vi "Write Header and Footer [ ].vi"(8 "error in (no error)":errorcluster, 10 "Header and Footer [ ]":T1, 11 "Header and Footer Class in":refnum<class "Header and Footer Class.lvclass">) -> (0 "error out":errorcluster, 3 "Header and Footer Class out":refnum<class "Header and Footer Class.lvclass">)   [LabVIEW 2020, in "Exaprom PDF.lvlib" / "Header and Footer Class.lvclass"]
uses:
  <userlib>/labview-PDF-writer-master/LV Class/Header and Footer Class/Header and Footer Class.lvclass
  <userlib>/labview-PDF-writer-master/LV Class/Header and Footer Class/VIs/Controls/Header Footer [ ] V2.ctl
  <userlib>/labview-PDF-writer-master/LV Class/Header and Footer Class/VIs/Controls/Header Footer cluster V2.ctl
  <userlib>/labview-PDF-writer-master/Controls/Header, Footer and Watermark Controls/Header or Footer.ctl
  <userlib>/labview-PDF-writer-master/Controls/Header, Footer and Watermark Controls/Header Footer Type.ctl
  <userlib>/labview-PDF-writer-master/Controls/Header, Footer and Watermark Controls/Header footer horiz alignment.ctl
  <userlib>/labview-PDF-writer-master/Controls/Table Controls/Cell Vertical alignment.ctl
  <userlib>/labview-PDF-writer-master/Controls/Text Controls/Line spacing.ctl
  <userlib>/labview-PDF-writer-master/Controls/Header, Footer and Watermark Controls/Page number.ctl
  <userlib>/labview-PDF-writer-master/Controls/Font Controls/Font complete cluster horizontal.ctl
  <userlib>/labview-PDF-writer-master/Controls/Font Controls/Font size.ctl
  <userlib>/labview-PDF-writer-master/Controls/Font Controls/Font color.ctl
  <userlib>/labview-PDF-writer-master/Controls/Font Controls/Type and encoding.ctl
  <userlib>/labview-PDF-writer-master/Controls/Text Controls/Unicode/Type and run direction.ctl
  C:/Program Files (x86)/National Instruments/LabVIEW 2020/user.lib/labview-PDF-writer-master/DLL/itextsharp.dll
  DLL/itextsharp.dll
  <userlib>/labview-PDF-writer-master/Controls/Header, Footer and Watermark Controls/Header Footer Line.ctl
  <userlib>/labview-PDF-writer-master/LV Class/Header and Footer Class/Header and Footer Class.lvclass/Header and Footer Class.ctl
  <userlib>/labview-PDF-writer-master/Exaprom PDF.lvlib
panel:
  # "X"
  # "Y"
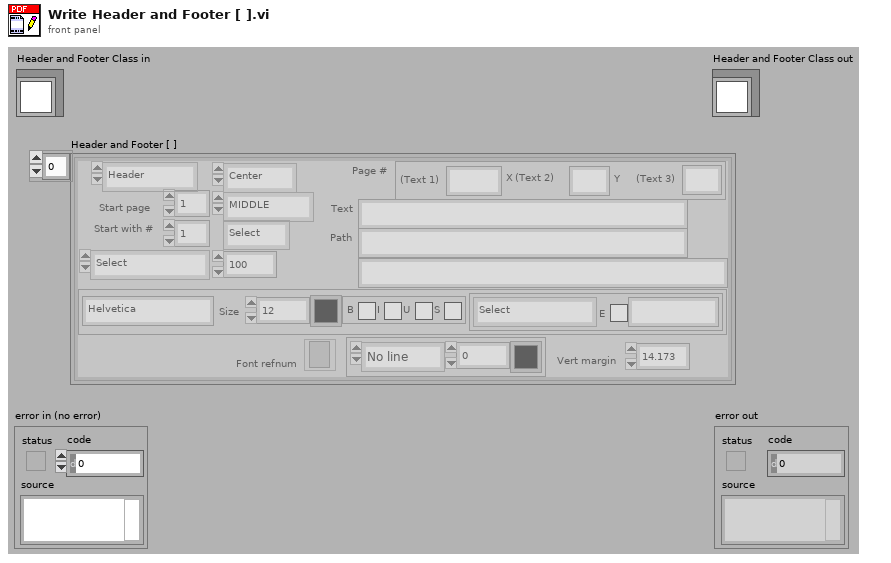
[diagram p1: front panel]
types:
  T1 = typedef "Exaprom PDF.lvlib/Header and Footer Class.lvclass/Header Footer [ ] V2.ctl" = T2[]
  T2 = typedef "Exaprom PDF.lvlib/Header and Footer Class.lvclass/Header Footer cluster V2.ctl" = cluster{"Header or Footer":T3, "Start page":i32, "Start with #":i32, "Type":T4, "Alignment":T5, "Vertical Alignement":T6, "Line spacing":T7, "Image (%)":sgl, "Page #":T8, "Text":string, "Path":string, "Font":T9, "Font refnum":refnum<k24>, "Line":cluster{"Line":T14, "Thickness (points)":sgl, "Colour":T11}, "Vert margin":dbl, "Hyperlink":string}
  T3 = typedef "Exaprom PDF.lvlib/Header or Footer.ctl" = enum16{"Header", "Footer"}
  T4 = typedef "Exaprom PDF.lvlib/Header Footer Type.ctl" = enum16{"Select", "Text", "Text + hyperlink", "Page number", "Image", "Image + hyperlink"}
  T5 = typedef "Exaprom PDF.lvlib/Header footer horiz alignment.ctl" = enum16{"Left", "Center", "Right"}
  T6 = typedef "Exaprom PDF.lvlib/Cell Vertical alignment.ctl" = enum16{"TOP", "MIDDLE", "BOTTOM"}
  T7 = typedef "Exaprom PDF.lvlib/Line spacing.ctl" = enum16{"Select", "1.0", "1.5", "2.0"}
  T8 = typedef "Exaprom PDF.lvlib/Page number.ctl" = cluster{"Text 1":string, "Text 2":string, "Text 3":string}
  T9 = typedef "Exaprom PDF.lvlib/Font complete cluster horizontal.ctl" = cluster{"Name":string, "Size":T10, "Color":T11, "Style":cluster{"Bold":bool, "Italic":bool, "Underline":bool, "Strikeout":bool}, "Type":T12}
  T10 = typedef "Exaprom PDF.lvlib/Font size.ctl" = sgl
  T11 = typedef "Exaprom PDF.lvlib/Font color.ctl" = u32
  T12 = typedef "Exaprom PDF.lvlib/Type and encoding.ctl" = cluster{"Type&direction":T13, "Embedded":bool, "Encoding":string}
  T13 = typedef "Exaprom PDF.lvlib/Type and run direction.ctl" = enum16{"Select", "ASCII", "UTF-16", "UTF-16 (default)", "UTF-16 (LTR)", "UTF-16 (RTL)"}
  T14 = typedef "Exaprom PDF.lvlib/Header Footer Line.ctl" = enum16{"No line", "Horizontal line"}
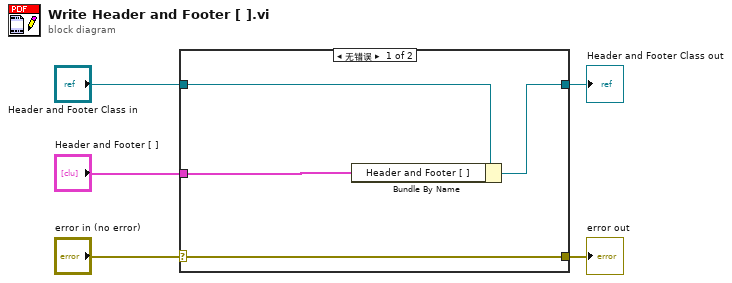
[diagram p0: block diagram]
diagram:
  n1 = case shown="无错误" "error in (no error)" {
    selector: "error in (no error)" -> [w9 w10]
    tunnel: [w9 w10] -> w4
    tunnel: [w7 w11] -> w2
    tunnel: "Header and Footer Class in" -> [w8 w11]
    tunnel: "Header and Footer [ ]" -> [w6 _]
    frame No Error {
      n2 = Bundle By Name(cluster=w8, "Header and Footer [ ]"=w6) -> (w7:refnum<class "Header and Footer Class.lvclass">)
    }
    frame Error {
    }
  }
  "error out" <- w4
  "Header and Footer Class out" <- w2
